vi "Enqueue Message (Single).vi"(6 "Nachricht mit Priorität? (F)":bool, 8 "error in (no error)":T1 caption="Fehler (Eingang, kein Fehler)", 9 "Nachrichtendaten":variant, 10 "Nachricht":string, 11 "Nachrichten-Queue":refnum<queue>) -> (0 "error out":T1 caption="Fehler (Ausgang)", 3 "Nachrichten-Queue (Kopie)":refnum<queue>)   [LabVIEW 2014, in "MyQH Message Queue.lvlib"]
doc: "Normale Nachrichten werden an die Queue angehängt. Nachrichten mit hoher Priorität werden an den Anfang der Queue eingefügt."
uses:
  MyQH Message Queue.lvlib
  Message Cluster.ctl
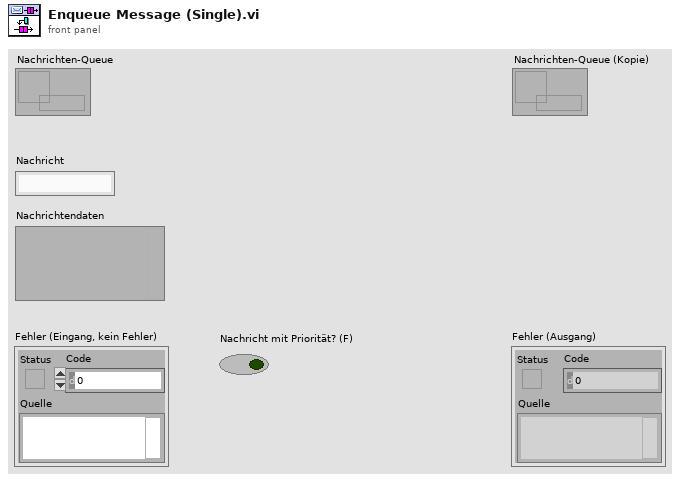
[diagram p1: front panel]
types:
  T1 = cluster{"Status":bool, "Code":i32, "Quelle":string}
  T2 = typedef "MyQH Message Queue.lvlib/Message Cluster.ctl" = cluster{"Nachricht":string, "Nachrichtendaten":variant}
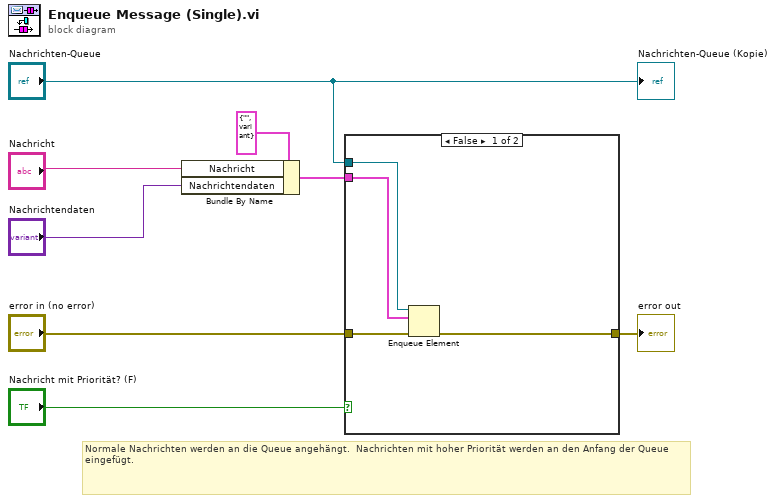
[diagram p0: block diagram]
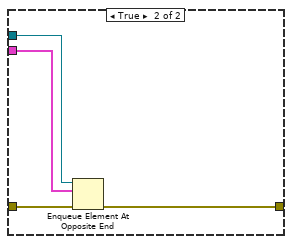
[diagram p2: hidden frame]
diagram:
  # "Normale Nachrichten werden an die Queue angehängt.  Nachrichten mit hoher Priorität werden an den Anfang der Queue eingefügt."
  n1 = Bundle By Name(cluster=T2 {"Nachricht"="", "Nachrichtendaten"=variant} ("Message Cluster"), "Nachricht"="Nachricht", "Nachrichtendaten"="Nachrichtendaten") -> (w1:T2)
  n2 = case shown="False" "Nachricht mit Priorität? (F)" {
    tunnel: "error in (no error)" -> [w12 w16]
    tunnel: [w11 w15] -> w3
    tunnel: "Nachrichten-Queue" -> [w10 w14]
    tunnel: w1 -> [w9 w13]
    frame False {
      n3 = Enqueue Element(queue=w10, element=w9, error in (no error)=w12) -> (error out=w11:errorcluster)  [unwired: 1 in, 2 out]
    }
    frame True {
      n4 = Enqueue Element At Opposite End(queue=w14, element=w13, error in (no error)=w16) -> (error out=w15:errorcluster)  [unwired: 1 in, 2 out]
    }
  }
  "error out" <- w3
  "Nachrichten-Queue (Kopie)" <- "Nachrichten-Queue"
